vi "Destroy.vi"(8 "error in (no error)":errorcluster, 10 "Shared Key":string, 11 "SMO":refnum<class "SMO.lvclass">) -> (0 "error out":errorcluster)   [LabVIEW 2013, in "SMO.lvclass"]
doc: "Destructor\n\nNote 01: This method is overridable by descendant\nNote 02: When overridden, Call Parent Method is required\n\n---------------------------------------------------------------\nJKI State Machine Objects™\nhttp://jki.net/state-machine-objects/\nCopyright (C) 2005-2015, JKI <info@jki.net>\nALL RIGHTS RESERVED"
uses:
  SMO.lvclass
  Typedefs/SMOState --Enum.ctl
  SMO.lvclass/SMO.ctl
  Registry/Registry-SMO.lvclass
panel:
  # "For instructions on how to use the JKI State Machine Objects, examples and video tutorials, visit:\nhttp://jki.net/state-machine-objects/\n\nJKI State Machine Objects™\nhttp://jki.net/state-machine-objects/\nCopyright (C) 2005-2015, JKI <info@jki.net>\nALL RIGHTS RESERVED"
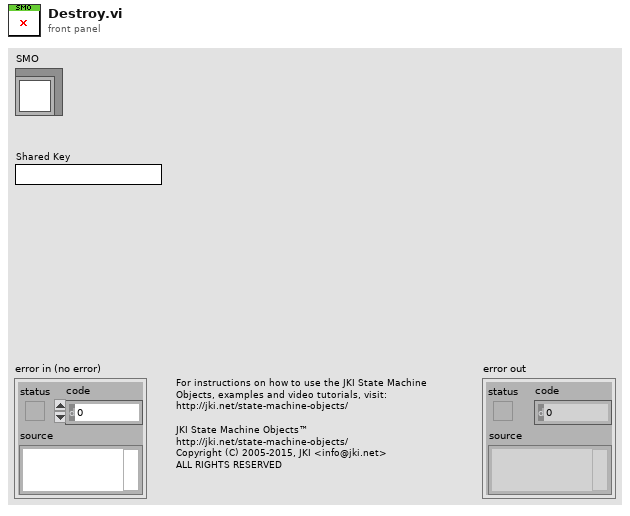
[diagram p1: front panel]
types:
  T1 = typedef "SMO.lvclass/SMOState --Enum.ctl" = enum16{"unknown", "Created", "Started", "Stopped"}
  T2 = typedef "SMO.lvclass/Public Events.ctl" = cluster{"Error":refnum<user-event>, "State":refnum<user-event>, "Reserve State":refnum<user-event>}
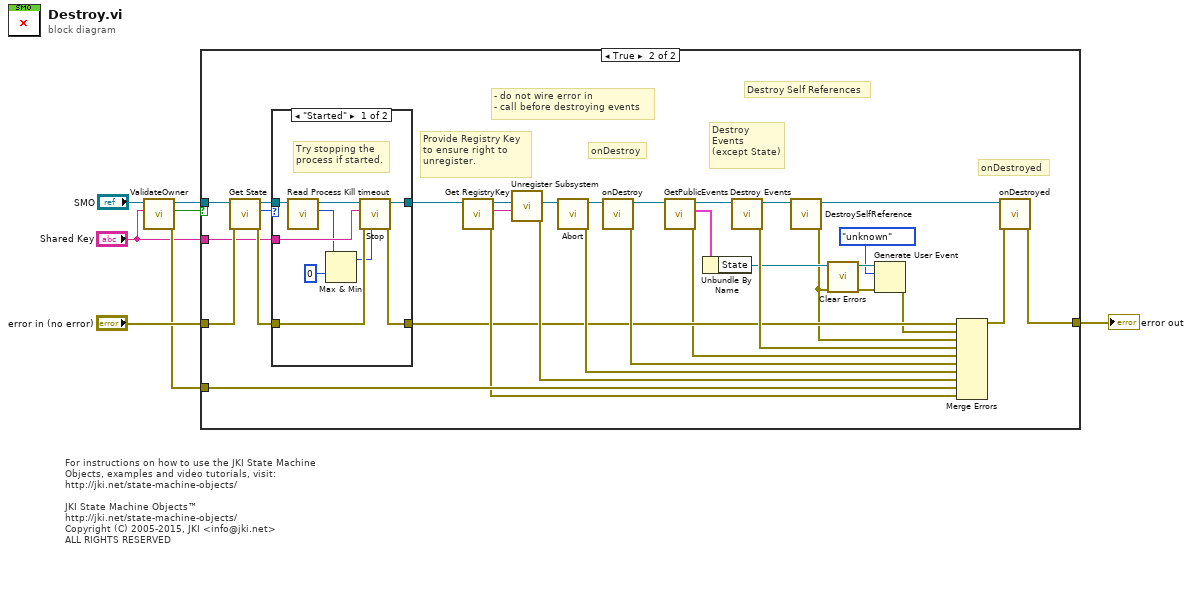
[diagram p0: block diagram]
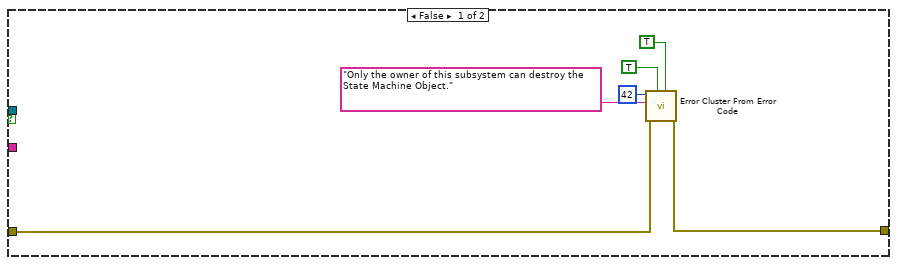
[diagram p2: hidden frame]
diagram:
  # "For instructions on how to use the JKI State Machine Objects, examples and video tutorials, visit:\nhttp://jki.net/state-machine-objects/\n\nJKI State Machine Objects™\nhttp://jki.net/state-machine-objects/\nCopyright (C) 2005-2015, JKI <info@jki.net>\nALL RIGHTS RESERVED"
  n1 = call "ValidateOwner.vi"("Shared Key"="Shared Key", "SMO in"="SMO") -> ("error out"=w3:errorcluster, "key matched"=w2:bool, "SMO out"=w4:refnum<class "SMO.lvclass">)  [unwired: 7 in]
  n2 = case shown="True" w2 {
    tunnel: "error in (no error)" -> [w10 w29]
    tunnel: [w9 w40] -> w6
    tunnel: w4 -> [_ w30]
    tunnel: w3 -> [_ w39]
    tunnel: "Shared Key" -> [_ w23]
    frame False {
      n3 = call <vilib>:"Error Cluster From Error Code.vi"("is warning? (False)"=TRUE, "show call chain? (False)"=TRUE, "error in (no error)"=w10, "error message (\"\")"="Only the owner of this subsystem can destroy the State Machine Object." ("error message (\"\")"), "error code (0)"=42) -> ("error out"=w9:errorcluster)  [unwired: 4 in]
    }
    frame True {
      # "Provide Registry Key\nto ensure right to \nunregister."
      # "Destroy\nEvents\n(except State)"
      # "Destroy Self References"
      # "onDestroy"
      # "onDestroyed"
      # "- do not wire error in\n- call before destroying events"
      n4 = call "Get State.vi"("error in (no error)"=w29, "SMO"=w30) -> ("error out"=w24:errorcluster, "SMO State"=w28:T1, "SMO out"=w27:refnum<class "SMO.lvclass">)  [unwired: 7 in]
      n5 = case shown="\"Started\"" w28 {
        tunnel: w27 -> [w49 w55]
        tunnel: [w52 w55] -> w26
        tunnel: [w50 w54] -> w25
        tunnel: w24 -> [w51 w54]
        tunnel: w23 -> [w53 _]
        frame "Started" {
          # "Try stopping the\nprocess if started."
          n6 = call "Read Process Kill timeout.vi"("SMO in"=w49) -> ("Process Kill timeout (ms)"=w47:i32, "SMO out"=w48:refnum<class "SMO.lvclass">)  [unwired: 9 in]
          n7 = Max & Min(x=w47, y=0) -> (max(x,y)=w46:i32)  [unwired: 1 out]
          n8 = call "Stop.vi"("timeout in ms (-1)"=w46, "error in (no error)"=w51, "Shared Key"=w53, "SMO"=w48) -> ("error out"=w50:errorcluster, "SMO out"=w52:refnum<class "SMO.lvclass">)  [unwired: 6 in]
        }
        frame Default {
        }
      }
      n9 = call "Get RegistryKey.vi"("SMO"=w26) -> ("error out"=w31:errorcluster, "RegistryKey"=w32:string, "SMO out"=w33:refnum<class "SMO.lvclass">)  [unwired: 8 in]
      n10 = call "Unregister Subsystem.vi"("RegistryKey"=w32, "JKI SMO"=w33) -> ("error out"=w42:errorcluster, "JKI SMO out"=w44:refnum<class "SMO.lvclass">)  [unwired: 8 in]
      n11 = call "Abort.vi"("SMO"=w44) -> ("error out"=w43:errorcluster, "SMO out"=w37:refnum<class "SMO.lvclass">)  [unwired: 9 in]
      n12 = call-dynamic "onDestroy.vi"("SMO"=w37) -> ("error out"=w35:errorcluster, "SMO out"=w22:refnum<class "SMO.lvclass">)  [unwired: 9 in]
      n13 = call "GetPublicEvents.vi"("SMO"=w22) -> ("error out"=w20:errorcluster, "Public Events"=w19:T2, "SMO out"=w21:refnum<class "SMO.lvclass">)  [unwired: 8 in]
      n14 = Unbundle By Name(w19) -> ("State"=w18:refnum<user-event>)
      n15 = call "Destroy Events.vi"("SMO"=w21) -> ("error out"=w34:errorcluster, "SMO out"=w36:refnum<class "SMO.lvclass">)  [unwired: 9 in]
      n16 = call-dynamic "DestroySelfReference.vi"("SMO"=w36) -> ("error out"=w14:errorcluster, "SMO out"=w38:refnum<class "SMO.lvclass">)  [unwired: 9 in]
      n17 = call <vilib>:"Clear Errors.vi"("error in (no error)"=w14) -> ("error out"=w15:errorcluster)  [unwired: 6 in]
      n18 = Generate User Event(user event=w18, event data cluster=SMOState_--Enum."unknown" ("event data"), error in=w15) -> (error out=w16:errorcluster)  [unwired: 1 in, 1 out]
      n19 = Merge Errors(w25, w16, w14, w34, w20, w35, w43, w42, w39, w31) -> (w41:errorcluster)
      n20 = call-dynamic "onDestroyed.vi"("error in (no error)"=w41, "SMO"=w38) -> ("error out"=w40:errorcluster)  [unwired: 9 in]
    }
  }
  "error out" <- w6
